vi "labview_files.vi"() -> ()   [LabVIEW 2020]
uses:
  <vilib>/Platform/TimedLoop/XDataNode/timing_clust.ctl
  <vilib>/Platform/TimedLoop/XDataNode/nitl_modes.ctl
  <vilib>/Platform/TimedLoop/XDataNode/wakeup.ctl
  <vilib>/Utility/NIReport.llb/Report Type.ctl
  <vilib>/Instr/_visa.llb/VISA Configure Serial Port (Instr).vi
  <vilib>/Utility/NIReport.llb/Append Text Table to Report (wrap).vi
  <vilib>/platform/TimedLoop/XDataNode/XDataNode.xnode
  <vilib>/Utility/NIReport.llb/NI_report.lvclass
  <vilib>/Utility/NIReport.llb/NI_ReportGenerationCore.lvlib
  <vilib>/Utility/NIReport.llb/Excel/NI_Excel.lvclass
  <vilib>/Platform/TimedLoop/XDataNode/XDNodeRunTimeDep.lvlib
panel:
  out "Mea_Rows":string[](array[string])=["Pin Status", "Variable Name", "Var. Status", "Inverse"]
  in  "stop":bool
  in  "input 3":dbl
  in  "input 4":dbl
  out "AVR Speed":dbl
  out "SUM Speed":dbl
  in  "report file path 3":path
  in  "General Control":T1(tab)
  out "FREE_MODE_LED":bool
  out "CYCLE_MODE_LED":bool
  out "OFF_RECORD":bool
  out "ON_RECORD":bool
  out "count_mea_time":dbl
  in  "RECORDER":bool
  out "Amperage of Battery":dbl
  out "Voltage of Battery":dbl
  out "Angular Speed III":dbl
  out "Torque III":dbl
  in  "FREE/CYCLE":bool
  out "Speed of Wheel":dbl
  out "Voltage of Genarator":dbl
  out "Set Speed":dbl
  out "Setponit_V":dbl
  out "Angular Speed II":dbl
  out "Angular Speed I":dbl
  in  "START":bool
  in  "Notice":enum32{"Massage", "Measurement", "demo"}(tab)
  out "Message":string[][](array[string])
  out "Measurement":string[][](array[string])
  out "demooo":string[][](array[string])
  in  "MEASURE":bool
  in  "Plot":enum32{"SPEED", "TORQUE", "ANGULAR SPEED"}(tab)
  out "SCOPE_SPEED":dynamicdata(graph)
  out "SCOPE_TORQUE":dynamicdata(graph)
  out "SCOPE_AS":dynamicdata(graph)
  in  "(KM/H)":dbl(knob) scale=0.0..50.0
  in  "?":bool
  out "Torque II":dbl
  out "Torque I":dbl
  in  "Measurement time (s)":dbl=1.0 min=0.0 max=1500.0
  in  "VISA resource name":refnum<visa-resource-name>
  out "Fcan":dbl
  out "Fa":dbl
  out "FDr":dbl
  out "FR":dbl
  in  "Service":T2(tab)
  in  "inv1_AI1":dbl
  # "Electric Vehicle Powertrain System Education Model"
  # "MEASUREMENT"
  # "CHOOSE MODE"
  # "SET SPEED"
  # "CONTROL"
  # "RECORDER"
  # "ON"
  # "CYCLE"
  # "FREE"
  # "OFF"
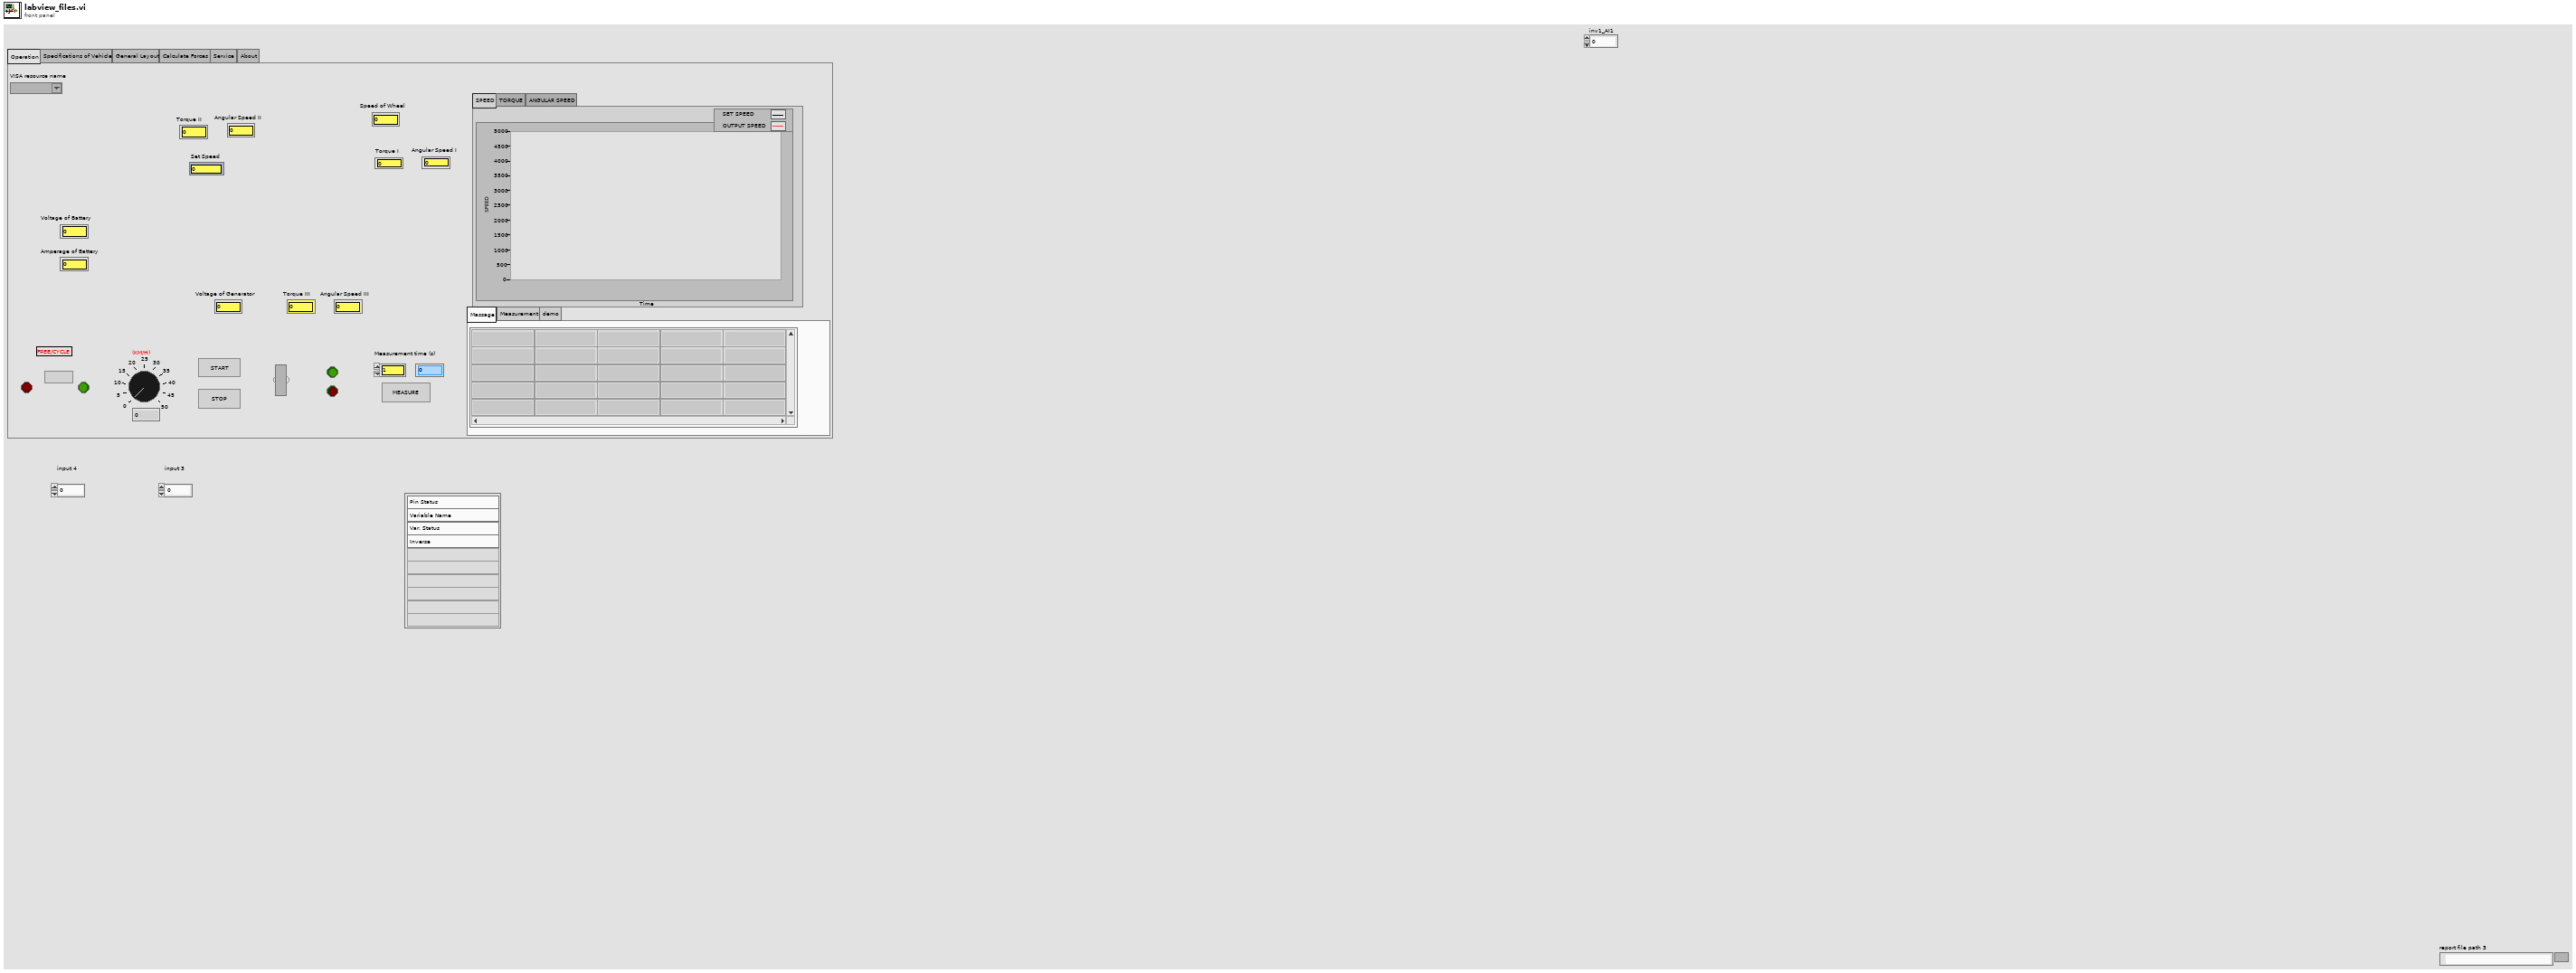
[diagram p1: front panel]
types:
  T1 = enum32{"Operation", "Specifications of Vehicle", "General Layout", "Calculate Forces", "Service", "About"}
  T2 = enum32{"Calib Loadcell of Generator", "Calib Loadcell of Motor", "Moment of  Bench", "Forces on Model", "Encoder", "PID Specifications"}
  T3 = typedef "XDNodeRunTimeDep.lvlib/timing_clust.ctl" = cluster{"Expected End [f-1]":u64, "Actual End [f-1]":u64, "Finished Late? [f-1]":bool, "Expected End [i-1]":u64, "Actual End [i-1]":u64, "Finished Late? [i-1]":bool, "Expected Start [i]":u64, "Actual Start [i]":u64, "Expected Start [f]":u64, "Actual Start [f]":u64, "Source Name":string, "Structure Name":string, "Period":i64, "Deadline":i64, "Offset":i64, "Start":i64, "Priority":i32, "Timeout":i32, "Mode":T4, "Wakeup Reason":T5, "Error":errorcluster, "Source Type":string, "Secondary Source Type":string, "Global End Time":u64, "Global Start Time":u64, "Frame Duration":u64, "Iteration Duration":u64, "Assigned CPU":i32, "I/O Scan Engine Mode":u32}
  T4 = typedef "XDNodeRunTimeDep.lvlib/nitl_modes.ctl" = enum32{"No Change", "Process missed periods, maintain original phase", "Discard missed periods, maintain original phase", "Process missed periods, ignore original phase", "Discard missed periods, ignore original phase"}
  T5 = typedef "XDNodeRunTimeDep.lvlib/wakeup.ctl" = enum32{"Normal", "Aborted", "Asynchronous wakeup", "Timing source error", "Timed loop error", "Timeout"}
  T6 = typedef "NI_ReportGenerationCore.lvlib/Report Type.ctl" = enum16{"HTML", "Word", "Excel"}
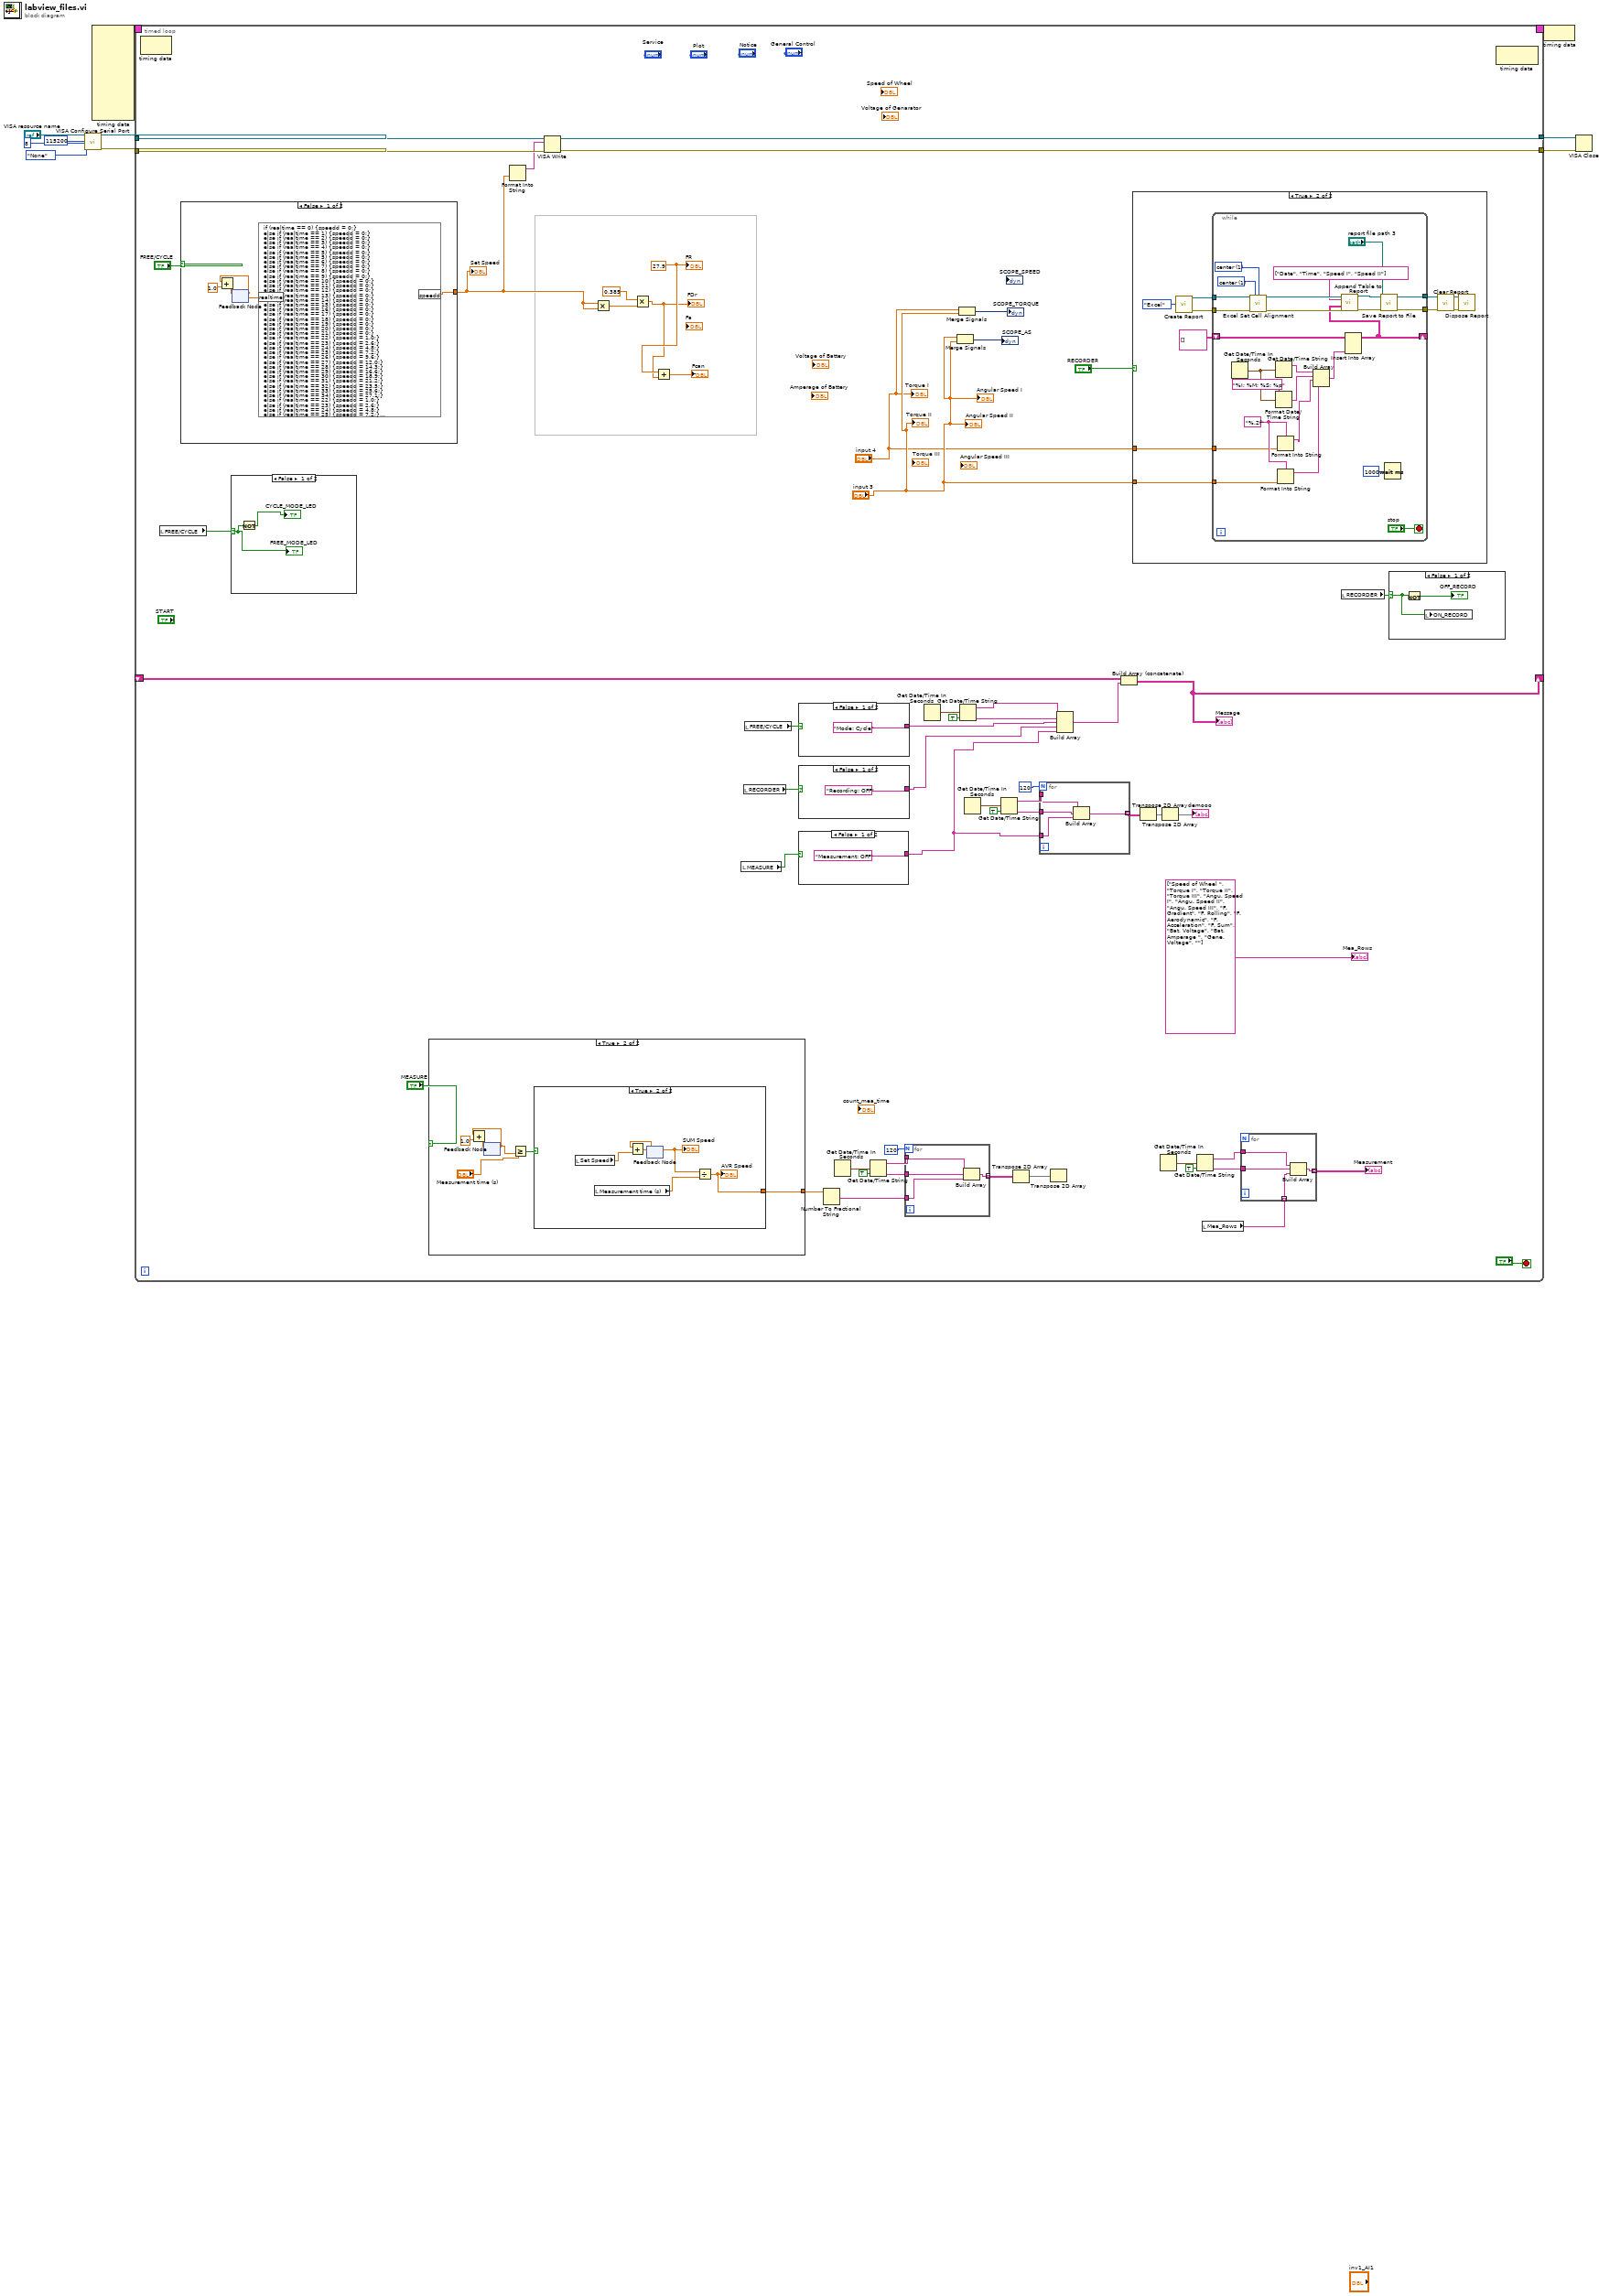
[diagram p0: block diagram]
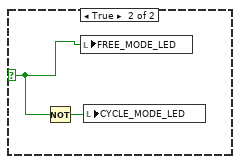
[diagram p2: hidden frame]
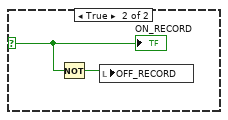
[diagram p3: hidden frame]
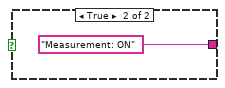
[diagram p4: hidden frame]
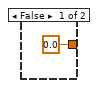
[diagram p5: hidden frame]
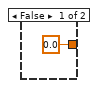
[diagram p6: hidden frame]
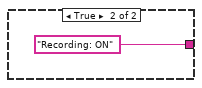
[diagram p7: hidden frame]
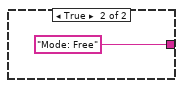
[diagram p8: hidden frame]
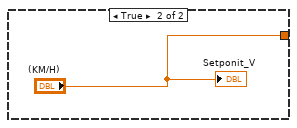
[diagram p9: hidden frame]
diagram:
  n1 = call-poly "VISA Configure Serial Port"("VISA resource name"="VISA resource name", "baud rate (9600)"=u32 115200, "data bits (8)"=u16 8, "parity (0:none)"=enum16{"None", "Odd", "Even", "Mark", "Space"}."None") -> ("VISA resource name out"=w4:refnum<visa-resource-name>, "error out"=w3:errorcluster)  [unwired: 10 in]
  n2 = node-c288() -> (w10:T3)  [unwired: 10 in]
  n3 = timed-loop {
    timing: w10 -> [_]
    timing-out: [_] -> w9
    tunnel: w4 -> [w60]
    tunnel: w3 -> [w59]
    tunnel: [w58] -> w2
    tunnel: [w57] -> w1
    shift-right: [w21] -> _
    shift-left: _ -> [w20]
    stop <- "?" stop-if-true
    w62 = 27.9 ("FR")
    n4 = node-c288() -> ()  [unwired: 1 in, 1 out]
    n5 = local read "FREE/CYCLE"() -> (w11:bool)
    n6 = case shown="False" "FREE/CYCLE" {
      tunnel: [w111 "(KM/H)"] -> w50
      frame False {
        n7 = feedback #1() -> (w108:dbl)  [unwired: 1 in]
        n8 = Add(x=w108, y=1.0) -> (x+y=w109:dbl)
        n9 = feedback-in #1(w109) -> ()
        n10 = formula code="if (realtime == 0) {speedd = 0;}\nelse if (realtime == 1) {speedd = 0;}\nelse if (realtime == 2) {speedd = 0;}\nelse if (realtime == 3) {speedd = 0;}\nelse if (realtime == 4) {speedd = 0;}\nelse if (realtime == 5) {speedd = 0;}\nelse if (realtime == 5) {speedd = 0;}\nelse if (realtime == 6) {speedd = 0;}\nelse if (realtime == 7) {speedd = 0;}\nelse if (realtime == 8) {speedd = 0;}\nelse if (realtime == 9) {speedd = 0;}\nelse if (realtime == 10) {speedd = 0;}\nelse if (realtime == 11) {speedd = 0;}\nelse if (realtime == 12) {speedd = 0;}\nelse if (realtime == 13) {speedd = 0;}\nelse if (realtime == 14) {speedd = 0;}\nelse if (realtime == 15) {speedd = 0;}\nelse if (realtime == 16) {speedd = 0;}\nelse if (realtime == 17) {speedd = 0;}\nelse if (realtime == 18) {speedd = 0;}\nelse if (realtime == 19) {speedd = 0;}\nelse if (realtime == 20) {speedd = 0;}\nelse if (realtime == 21) {speedd = 0;}\nelse if (realtime == 22) {speedd = 1.0;}\nelse if (realtime == 23) {speedd = 2.6;}\nelse if (realtime == 24) {speedd = 4.8;}\nelse if (realtime == 25) {speedd = 7.2;}\nelse if (realtime == 26) {speedd = 9.6;}\nelse if (realtime == 27) {speedd = 12.0;}\nelse if (realtime == 28) {speedd = 14.3;}\nelse if (realtime == 29) {speedd = 16.6;}\nelse if (realtime == 30) {speedd = 18.9;}\nelse if (realtime == 31) {speedd = 21.2;}\nelse if (realtime == 32) {speedd = 23.5;}\nelse if (realtime == 33) {speedd = 25.6;}\nelse if (realtime == 34) {speedd = 27.1;}\nelse if (realtime == 22) {speedd = 1.0;}\nelse if (realtime == 23) {speedd = 2.6;}\nelse if (realtime == 24) {speedd = 4.8;}\nelse if (realtime == 25) {speedd = 7.2;}\nelse if (realtime == 26) {speedd = 9.6;}\nelse if (realtime == 27) {speedd = 12.0;}\nelse if (realtime == 28) {speedd = 14.3;}\nelse if (realtime == 29) {speedd = 16.6;}\nelse if (realtime == 30) {speedd = 18.9;}\nelse if (realtime == 31) {speedd = 21.2;}\nelse if (realtime == 32) {speedd = 23.5;}\nelse if (realtime == 33) {speedd = 25.6;}\nelse if (realtime == 34) {speedd = 27.1;}\nelse if (realtime == 35) {speedd = 28.0;}\nelse if (realtime == 36) {speedd = 28.7;}\nelse if (realtime == 37) {speedd = 29.2;}\nelse if (realtime == 38) {speedd = 29.8;}\nelse if (realtime == 39) {speedd = 30.3;}\nelse if (realtime == 40) {speedd = 29.6;}\nelse if (realtime == 41) {speedd = 28.7;}\nelse if (realtime == 42) {speedd = 27.9;}\nelse if (realtime == 43) {speedd = 27.5;}\nelse if (realtime == 44) {speedd = 27.3;}\nelse if (realtime == 45) {speedd = 27.3;}\nelse if (realtime == 46) {speedd = 27.4;}\nelse if (realtime == 47) {speedd = 27.5;}\nelse if (realtime == 48) {speedd = 27.6;}"("realtime"=w108) -> ("speedd"=w111:dbl)
      }
      frame True {
        "Setponit_V" <- "(KM/H)"
      }
    }
    "Set Speed" <- w50
    n11 = case shown="False" w11 {
      selector: w11 -> [w69 w71]
      frame False {
        n12 = Not(x=w69) -> (.not. x?=→"CYCLE_MODE_LED":bool)
        "FREE_MODE_LED" <- w69
      }
      frame True {
        n13 = Not(x=w71) -> (.not. x?=w72:bool)
        n14 = local write "FREE_MODE_LED"(w71) -> ()
        n15 = local write "CYCLE_MODE_LED"(w72) -> ()
      }
    }
    n16 = case shown="True" "MEASURE" {
      tunnel: [0.0 w88] -> w37
      frame False {
      }
      frame True {
        n17 = feedback #2() -> (w91:dbl)  [unwired: 1 in]
        n18 = Add(x=w91, y=1.0) -> (x+y=w92:dbl)
        n19 = feedback-in #2(w92) -> ()
        n20 = Greater Or Equal?(x=w91, y="Measurement time (s)") -> (x >= y?=w89:bool)
        n21 = case shown="True" w89 {
          tunnel: [0.0 w95] -> w88
          frame False {
          }
          frame True {
            n22 = local read "Set Speed"() -> (w99:dbl)
            n23 = local read "Measurement time (s)"() -> (w96:dbl)
            n24 = feedback #3() -> (w97:dbl)  [unwired: 1 in]
            "SUM Speed" <- w97
            n25 = Add(x=w97, y=w99) -> (x+y=w98:dbl)
            n26 = feedback-in #3(w98) -> ()
            n27 = Divide(x=w97, y=w96) -> (x/y=w95:dbl)
            "AVR Speed" <- w95
          }
        }
      }
    }
    n28 = Format Into String(w50) -> (resulting string=w56:string)  [unwired: 3 in, 1 out]
    n29 = VISA Write(VISA resource name=w60, write buffer=w56, error in (no error)=w59) -> (VISA resource name out=w58:refnum<visa-resource-name>, error out=w57:errorcluster)  [unwired: 1 out]
    n30 = Multiply(x=w50, y=w50) -> (x*y=w64:dbl)
    n31 = Multiply(x=0.385, y=w64) -> (x*y=w61:dbl)
    "FDr" <- w61
    n32 = Add(x=w62, y=w61) -> (x+y=→"Fcan":dbl)
    n33 = local read "MEASURE"() -> (w35:bool)
    n34 = local read "RECORDER"() -> (w33:bool)
    n35 = local read "FREE/CYCLE"() -> (w48:bool)
    n36 = case shown="False" w35 {
      tunnel: ["Measurement: OFF" ("element") "Measurement: ON" ("element")] -> w27
      frame False {
      }
      frame True {
      }
    }
    n37 = case shown="False" w48 {
      tunnel: ["Mode: Cycle" ("element") "Mode: Free" ("element")] -> w47
      frame False {
      }
      frame True {
      }
    }
    n38 = case shown="False" w33 {
      tunnel: ["Recording: OFF" ("element") "Recording: ON" ("element")] -> w46
      frame False {
      }
      frame True {
      }
    }
    n39 = Number To Fractional String(number=w37) -> (F-format string=w36:string)  [unwired: 3 in]
    n40 = Get Date/Time In Seconds() -> (seconds since 1Jan1904=w44:timestamp)
    n41 = Get Date/Time String(seconds (now)=w44, want seconds? (F)=TRUE) -> (date string=w42:string, time string=w41:string)  [unwired: 1 in]
    n42 = for {
      N: 120 -> [_]
      tunnel: [w103] -> w40 mode=indexing
      tunnel: w42 -> [w102]
      tunnel: w41 -> [w101]
      tunnel: w36 -> [w100]
      n43 = Build Array(w102, w101, w100) -> (w103:string[])
    }
    n44 = Get Date/Time In Seconds() -> (seconds since 1Jan1904=w54:timestamp)
    n45 = Merge Signals("input 3", "input 3") -> (→"SCOPE_AS":dynamicdata)
    n46 = Merge Signals("input 4", "input 3") -> (→"SCOPE_TORQUE":dynamicdata)
    n47 = Get Date/Time String(seconds (now)=w54, want seconds? (F)=TRUE) -> (date string=w52:string, time string=w51:string)  [unwired: 1 in]
    n48 = Get Date/Time In Seconds() -> (seconds since 1Jan1904=w32:timestamp)
    n49 = Get Date/Time String(seconds (now)=w32, want seconds? (F)=TRUE) -> (date string=w30:string, time string=w29:string)  [unwired: 1 in]
    n50 = Transpose 2D Array(2D array=w40) -> (transposed array=w23:string[][])
    n51 = for {
      N: 120 -> [_]
      tunnel: w30 -> [w84]
      tunnel: w29 -> [w83]
      tunnel: w27 -> [w82]
      tunnel: [w81] -> w26 mode=indexing
      n52 = Build Array(w84, w83, w82) -> (w81:string[])
    }
    n53 = Transpose 2D Array(2D array=w23) -> ()  [unwired: 1 out]
    n54 = Build Array(w52, w51, w47, w46, w27) -> (w22:string[])
    n55 = Build Array (concatenate)(w20, w22) -> (w21:string[][])
    "Message" <- w21
    n56 = case shown="True" "RECORDER" {
      tunnel: "input 4" -> [_ w114]
      tunnel: "input 3" -> [_ w113]
      frame False {
      }
      frame True {
        n57 = call <vilib>:"Create Report.vi"("report type"=Report_Type."Excel") -> ("report out"=w122:refnum<class "NI_report.lvclass">, "error out"=w121:errorcluster)  [unwired: 13 in]
        n58 = while {
          tunnel: w122 -> [w148]
          tunnel: w121 -> [w147]
          tunnel: [w139] -> w119
          tunnel: [w138] -> w118
          shift-right: [w132] -> _
          shift-left: string[][] [] -> [w133]
          tunnel: w114 -> [w129]
          tunnel: w113 -> [w128]
          stop <- "stop" stop-if-true
          w135 = "%.2f" ("format string")
          w145 = 1 items=["left", "center", "right"] ("horizontal alignment (left)")
          w146 = 1 items=["top", "center", "bottom"] ("vertical alignment (top)")
          n59 = Get Date/Time In Seconds() -> (seconds since 1Jan1904=w137:timestamp)
          n60 = call <vilib>:"Excel Set Cell Alignment.vi"("report in"=w148, "vertical alignment (top)"=w146, "horizontal alignment (left)"=w145, "error in (no error)"=w147) -> ("report out"=w144:refnum<class "NI_report.lvclass">, "error out"=w143:errorcluster)  [unwired: 10 in]
          n61 = Format Date/Time String(time format string (%c)="%I; %M; %S; %p", seconds (now)=w137) -> (date/time string=w126:string)  [unwired: 1 in]
          n62 = Get Date/Time String(seconds (now)=w137) -> (date string=w127:string)  [unwired: 2 in, 1 out]
          n63 = Format Into String(format string=w135, w129) -> (resulting string=w125:string)  [unwired: 2 in, 1 out]
          n64 = Format Into String(format string=w135, w128) -> (resulting string=w124:string)  [unwired: 2 in, 1 out]
          n65 = Build Array(w127, w126, w125, w124) -> (w134:string[])
          n66 = Insert Into Array(array=w133, new element=w134) -> (w132:string[][])  [unwired: 2 in]
          n67 = call-poly <vilib>:"Append Table to Report.vi"("report in"=w144, "column headers"=string[] ["Date", "Time", "Speed I", "Speed II"], "text data"=w132, "error in (no error)"=w143) -> ("report out"=w142:refnum<class "NI_report.lvclass">, "error out"=w141:errorcluster)  [unwired: 8 in, 2 out]
          n68 = call-dynamic "Save Report to File.vi"("report in"=w142, "report file path"="report file path 3", "error in (no error)"=w141) -> ("report out"=w139:refnum<class "NI_report.lvclass">, "error out"=w138:errorcluster)  [unwired: 11 in]
          n69 = Wait (ms)(milliseconds to wait=u32 1000) -> ()  [unwired: 1 out]
        }
        n70 = call-dynamic "Clear Report.vi"("report in"=w119, "error in (no error)"=w118) -> ("report out"=w117:refnum<class "NI_report.lvclass">, "error out"=w116:errorcluster)  [unwired: 12 in]
        n71 = call-dynamic "Dispose Report.vi"("report in"=w117, "error in (no error)"=w116) -> ()  [unwired: 13 in, 1 out]
      }
    }
    n72 = Transpose 2D Array(2D array=w26) -> (transposed array=w25:string[][])
    n73 = Get Date/Time In Seconds() -> (seconds since 1Jan1904=w17:timestamp)
    n74 = Transpose 2D Array(2D array=w25) -> (transposed array=→"demooo":string[][])
    n75 = Get Date/Time String(seconds (now)=w17, want seconds? (F)=TRUE) -> (date string=w15:string, time string=w14:string)  [unwired: 1 in]
    n76 = local read "Mea_Rows"() -> (w13:string[])
    n77 = for {
      tunnel: [w76] -> w12 mode=indexing
      tunnel: w13 -> [w75] mode=indexing
      tunnel: w15 -> [w74]
      tunnel: w14 -> [w73]
      n78 = Build Array(w74, w73, w75) -> (w76:string[])
    }
    "Measurement" <- w12
    n79 = local read "RECORDER"() -> (w19:bool)
    n80 = case shown="False" w19 {
      selector: w19 -> [w77 w80]
      frame False {
        n81 = Not(x=w77) -> (.not. x?=→"OFF_RECORD":bool)
        n82 = local write "ON_RECORD"(w77) -> ()
      }
      frame True {
        n83 = Not(x=w80) -> (.not. x?=w79:bool)
        n84 = local write "OFF_RECORD"(w79) -> ()
        "ON_RECORD" <- w80
      }
    }
    n85 = node-c288() -> ()  [unwired: 1 in, 1 out]
    "Torque I" <- "input 4"
    "Torque II" <- "input 3"
    "Angular Speed II" <- "input 3"
    "Angular Speed I" <- "input 3"
    "FR" <- w62
    "Mea_Rows" <- string[] ["Speed of Wheel ", "Torque I", "Torque II", "Torque III", "Angu. Speed I", "Angu. Speed II", "Angu. Speed III", "F. Gradient", "F. Rolling", "F.  Aerodynamic", "F. Acceleration", "F. Sum", "Bat. Voltage", "Bat. Amperage ", "Gene. Voltage", ""] ("Column Header Strings[]")
  }
  n86 = node-c288(w9) -> ()
  n87 = VISA Close(VISA resource name=w2, error in (no error)=w1) -> ()  [unwired: 1 out]
